vi "expand_image_horizontal.vi"(8 "error in (no error)":errorcluster, 10 "Expand By":i32, 11 "Image":T1) -> (0 "error out":errorcluster, 3 "Image Out":T1)   [LabVIEW 2016]
doc: "Expands an image in the horizontal direction. Old image sits in horizontal centre of new image."
uses:
  <vilib>/vision/Image Controls.llb/IMAQ Image.ctl
  <vilib>/vision/NI_Vision_Development_Module.lvlib
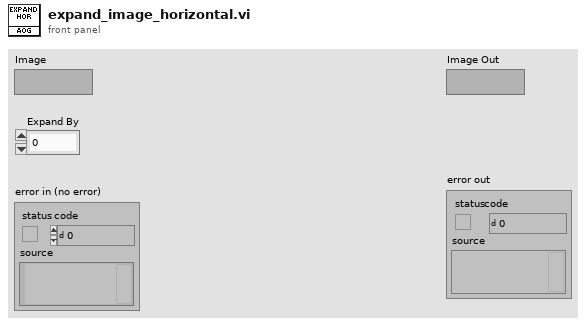
[diagram p1: front panel]
types:
  T1 = typedef "IMAQ Image.ctl" = refnum<image>
  T2 = typedef "Image Type" = u32
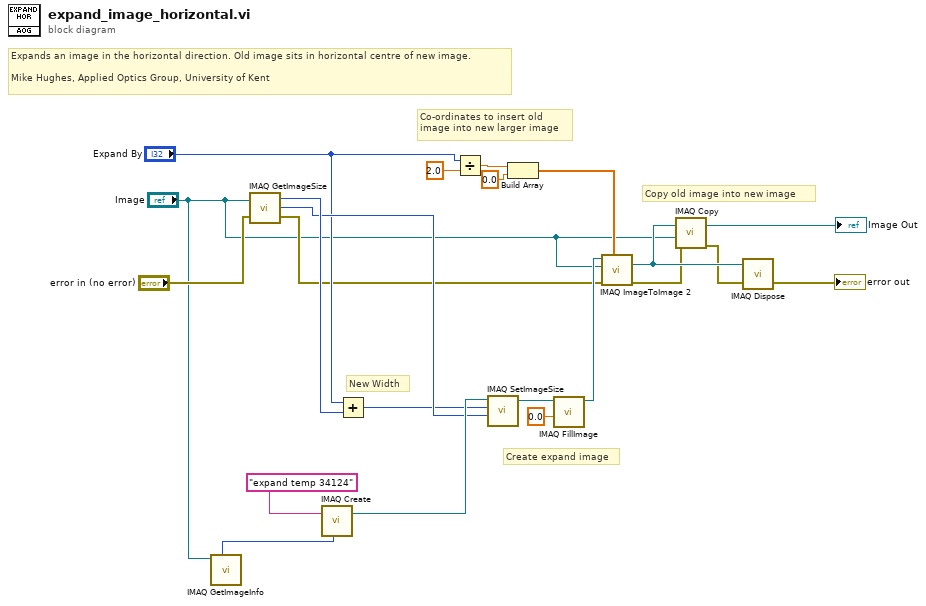
[diagram p0: block diagram]
diagram:
  # "Expands an image in the horizontal direction. Old image sits in horizontal centre of new image.\n\nMike Hughes, Applied Optics Group, University of Kent"
  # "Copy old image into new image"
  # "Create expand image"
  # "New Width"
  # "Co-ordinates to insert old \nimage into new larger image"
  n1 = call "IMAQ GetImageInfo"("Image"="Image") -> ("Image Type"=w2:T2)  [unwired: 3 in, 7 out]
  n2 = call "IMAQ GetImageSize"("Image"="Image", "error in (no error)"="error in (no error)") -> ("Y Resolution"=w15:i32, "X Resolution"=w20:i32, "error out"=w5:errorcluster)  [unwired: 2 in]
  n3 = call "IMAQ Create"("Image Name"="expand temp 34124", "Image Type"=w2) -> ("New Image"=w21:T1)  [unwired: 3 in, 1 out]
  n4 = Add(x="Expand By", y=w20) -> (x+y=w9:i32)
  n5 = Divide(x="Expand By", y=2.0) -> (x/y=w17:dbl)
  n6 = call "IMAQ SetImageSize"("Y Resolution"=w15, "X Resolution"=w9, "Image"=w21) -> ("Image Out"=w12:T1)  [unwired: 2 in, 1 out]
  n7 = Build Array(w17, 0.0 ("element")) -> (w16:dbl[])
  n8 = call "IMAQ FillImage"("Pixel Value (U8, U16, I16, Float)"=sgl 0.0, "Image"=w12) -> ("Image Out"=w10:T1)  [unwired: 8 in, 1 out]
  n9 = call "IMAQ ImageToImage 2"("Offset Left/Top"=w16, "error in (no error)"=w5, "Image Src (Small)"="Image", "Image Src (Large)"=w10) -> ("error out"=w4:errorcluster, "Image Dst Out"=w14:T1)  [unwired: 6 in]
  n10 = call "IMAQ Copy"("error in (no error)"=w4, "Image Dst"="Image", "Image Src"=w14) -> ("error out"=w13:errorcluster, "Image Dst Out"=→"Image Out":T1)  [unwired: 3 in]
  n11 = call "IMAQ Dispose"("Image"=w14, "error in (no error)"=w13) -> ("error out"=→"error out":errorcluster)  [unwired: 4 in]
